vi "Query Multi Eval Meas ACLR Limit Check Results.vi"(8 "error in (no error)":errorcluster, 9 "Result Type (Current)":i32(ring) items=["Current", "Average"], 10 "Instance (1)":T2=1, 11 "VISA resource name":refnum<visa-resource-name>) -> (0 "error out":errorcluster, 1 "ACLR Limit Check Results":T1, 2 "Reliability":i32, 3 "VISA resource name out":refnum<visa-resource-name>)   [LabVIEW 2015, in "Rohde&Schwarz CMXP NR FR2 Measurement.lvlib"]
doc: "Returns the multi eval measurement ACLR results.\n\nAttributes:\nRSCMXPNRFR2M_ATTR_QUERY_MULTI_EVAL_MEASUREMENT_ACLR_AVERAGE_LIMIT_CHECK_RESULTS\nRSCMXPNRFR2M_ATTR_QUERY_MULTI_EVAL_MEASUREMENT_ACLR_CURRENT_LIMIT_CHECK_RESULTS\n\nRemote-control commands:\nCALCulate:NRMMw:MEAS<i>:MEValuation:ACLR:AVERage?\nCALCulate:NRMMw:MEAS<i>:MEValuation:ACLR:CURRent?"
uses:
  <instrlib>/Rohde&Schwarz CMXP NR FR2 Measurement/Rohde&Schwarz CMXP NR FR2 Measurement.lvlib
  <instrlib>/Rohde&Schwarz CMXP NR FR2 Measurement/Private/_Instance.ctl
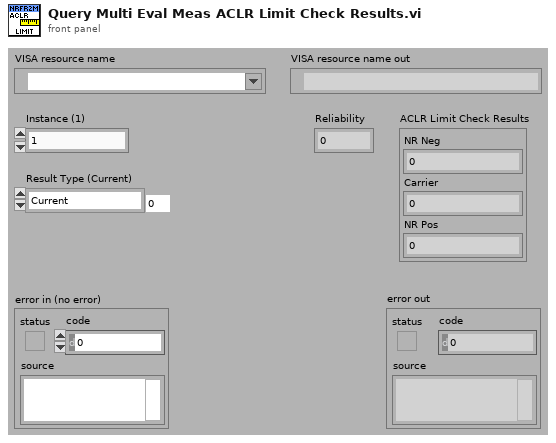
[diagram p1: front panel]
types:
  T1 = cluster{"NR Neg":i32, "Carrier":i32, "NR Pos":i32}
  T2 = typedef "Rohde&Schwarz CMXP NR FR2 Measurement.lvlib/_Instance.ctl" = i32
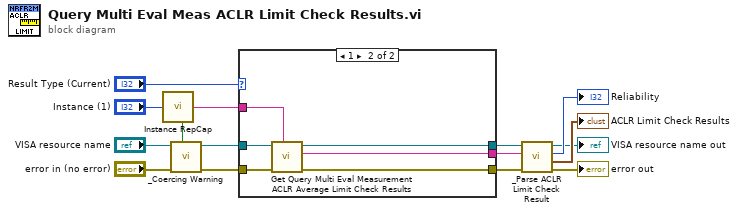
[diagram p0: block diagram]
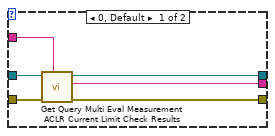
[diagram p2: hidden frame]
diagram:
  n1 = call <instrlib>:"Instance RepCap.vi"("Instance In"="Instance (1)") -> ("In Range?"=w2:bool, "RepCap Identifier Out"=w15:string)  [unwired: 1 in]
  n2 = call <instrlib>:"_Coercing Warning.vi"("In Range?"=w2, "error in (no error)"="error in (no error)", "VISA resource name"="VISA resource name") -> ("error out"=w3:errorcluster, "VISA resource name out"=w6:refnum<visa-resource-name>)  [unwired: 7 in]
  n3 = case shown="1" "Result Type (Current)" {
    tunnel: w3 -> [w20 w25]
    tunnel: w6 -> [w21 w24]
    tunnel: [w17 w23] -> w10
    tunnel: [w18 w22] -> w9
    tunnel: w15 -> [w19 w27]
    tunnel: [w16 w26] -> w13
    frame 0, Default {
      n4 = call "Get Query Multi Eval Measurement ACLR Current Limit Check Results"("Repeated Capabilities"=w19, "error in (no error)"=w20, "instrument handle"=w21) -> ("error out"=w17:errorcluster, "Query Multi Eval Measurement ACLR Current Limit Check Results"=w16:string, "instrument handle out"=w18:refnum<visa-resource-name>)  [unwired: 6 in]
    }
    frame 1 {
      n5 = call "Get Query Multi Eval Measurement ACLR Average Limit Check Results"("Repeated Capabilities"=w27, "error in (no error)"=w25, "instrument handle"=w24) -> ("error out"=w23:errorcluster, "Query Multi Eval Measurement ACLR Average Limit Check Results"=w26:string, "instrument handle out"=w22:refnum<visa-resource-name>)  [unwired: 6 in]
    }
  }
  n6 = call <instrlib>:"_Parse ACLR Limit Check Result.vi"("error in (no error)"=w10, "Input String"=w13, "VISA resource name"=w9) -> ("error out"=→"error out":errorcluster, "Limit Check Results"=→"ACLR Limit Check Results":T1, "Reliability"=→"Reliability":i32, "VISA resource name out"=→"VISA resource name out":refnum<visa-resource-name>)  [unwired: 5 in]
